vi "PCO_FFT.vi"(8 "error in (no error)":errorcluster, 11 "Data":dbl[][](graph)) -> (0 "error out":errorcluster, 3 "FFT":dbl[][](graph))   [LabVIEW 2026]
uses:
  <vilib>/Analysis/2dsp.llb/2D Real FFT.vi
  <vilib>/Analysis/NI_AALPro.lvlib
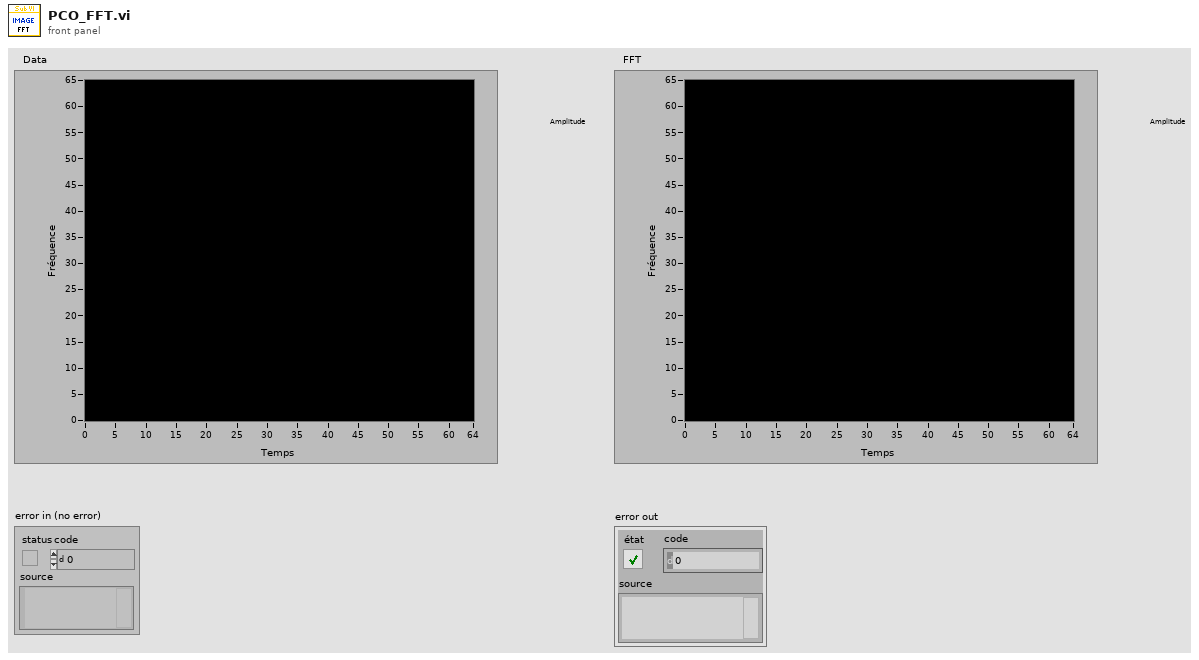
[diagram p1: front panel]
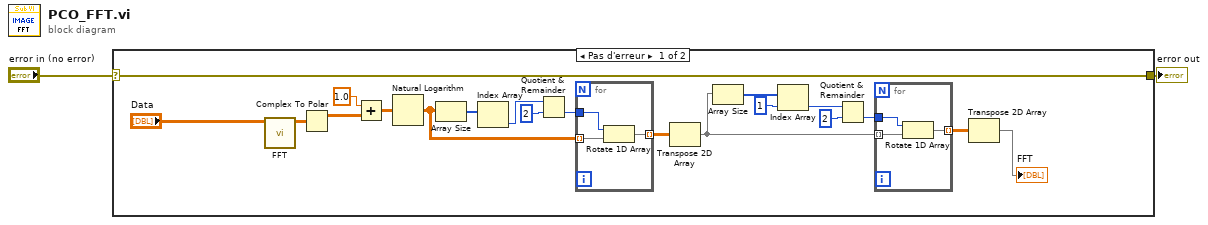
[diagram p0: block diagram]
diagram:
  n1 = case shown="Pas d'erreur" "error in (no error)" {
    selector: "error in (no error)" -> [w4 w29]
    tunnel: [w4 w29] -> w1
    frame No Error {
      n2 = call-poly <vilib>:"FFT.vi"("X"="Data") -> ("FFT {X}"=w22:cdb[][])  [unwired: 9 in, 1 out]
      n3 = Complex To Polar(r * e^(i*theta)=w22) -> (r=w20:dbl[][])  [unwired: 1 out]
      n4 = Add(x=1.0, y=w20) -> (x+y=w19:dbl[][])
      n5 = Natural Logarithm(1:w19) -> (0:w15:dbl[][])
      n6 = Array Size(array=w15) -> (size(s)=w18:i32[])
      n7 = Index Array(array=w18) -> (element=w17:i32)  [unwired: 1 in]
      n8 = Quotient & Remainder(x=w17, y=2) -> (floor(x/y)=w14:i32)  [unwired: 1 out]
      n9 = for {
        tunnel: w15 -> [w27] mode=indexing
        tunnel: w14 -> [w28]
        tunnel: [w26] -> w13 mode=indexing
        n10 = Rotate 1D Array(1:w27, 2:w28) -> (0:w26:dbl[])
      }
      n11 = Transpose 2D Array(2D array=w13) -> (transposed array=w8:dbl[][])
      n12 = Array Size(array=w8) -> (size(s)=w10:i32[])
      n13 = Index Array(array=w10, index=1 ("indice")) -> (element=w11:i32)
      n14 = Quotient & Remainder(x=w11, y=2) -> (floor(x/y)=w9:i32)  [unwired: 1 out]
      n15 = for {
        tunnel: w9 -> [w25]
        tunnel: w8 -> [w24] mode=indexing
        tunnel: [w23] -> w7 mode=indexing
        n16 = Rotate 1D Array(1:w24, 2:w25) -> (0:w23:dbl[])
      }
      n17 = Transpose 2D Array(2D array=w7) -> (transposed array=→"FFT":dbl[][])
    }
    frame Error {
    }
  }
  "error out" <- w1
